vi "Apply.vi"(8 "error in (no error)":errorcluster, 11 "IConfigure in":refnum<class "IConfigure.lvclass">) -> (0 "error out":errorcluster, 3 "IConfigure out":refnum<class "IConfigure.lvclass">)   [LabVIEW 2023, in "IConfigure.lvclass"]
uses:
  IConfigure.lvclass
  <vilib>/Utility/error.llb/Error Cluster From Error Code.vi
  <vilib>/ErrorRing/Error Ring.xnode
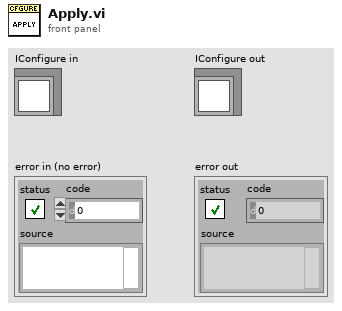
[diagram p1: front panel]
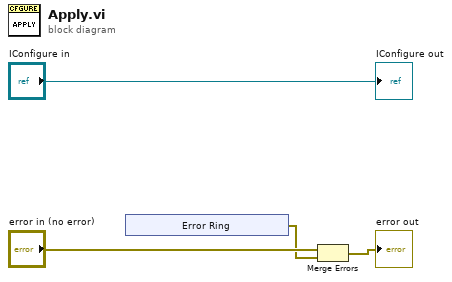
[diagram p0: block diagram]
diagram:
  n1 = xnode "Error Ring"() -> ("error out"=w1:errorcluster)
  n2 = Merge Errors("error in (no error)", w1) -> (→"error out":errorcluster)
  "IConfigure out" <- "IConfigure in"
